vi "Set Controlword.vi"(6 "Controlword":u8(ring), 7 "timeout (1s)":dbl=1.0 min=0.0, 8 "error in (no error)":errorcluster, 11 "SDO object in":refnum<k20>) -> (0 "error out":errorcluster, 1 "completion code":u32, 3 "SDO object out":refnum<k20>)   [LabVIEW 2016]
uses:
  <vilib>/CANopenLib/CANOPEN.llb/CANopen SDO Write [U16].vi
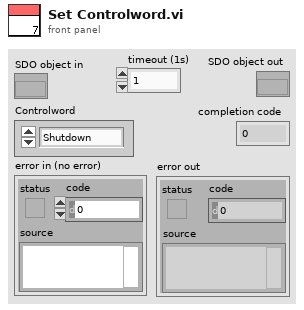
[diagram p1: front panel]
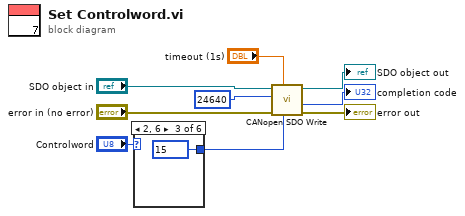
[diagram p0: block diagram]
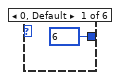
[diagram p2: hidden frame]
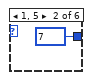
[diagram p3: hidden frame]
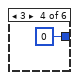
[diagram p4: hidden frame]
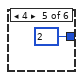
[diagram p5: hidden frame]
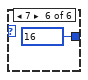
[diagram p6: hidden frame]
diagram:
  n1 = case shown="2, 6" "Controlword" {
    tunnel: [u16 6 u16 7 u16 15 u16 0 u16 2 u16 16] -> w7
    frame 0, Default {
    }
    frame 1, 5 {
    }
    frame 2, 6 {
    }
    frame 3 {
    }
    frame 4 {
    }
    frame 7 {
    }
  }
  n2 = call-poly <vilib>:"CANopen SDO Write.vi"("U16 data"=w7, "timeout (1s)"="timeout (1s)", "error in (no error)"="error in (no error)", "object index"=u16 24640, "SDO object in"="SDO object in") -> ("error out"=→"error out":errorcluster, "completion code"=→"completion code":u32, "SDO object out"=→"SDO object out":refnum<k20>)  [unwired: 4 in]
